vi "PDC_GetStatus.vi"(8 "error in (no error)":errorcluster, 11 "DeviceNo":u32) -> (0 "error out":errorcluster, 2 "Status":u32, 3 "ReturnValue":u32, 4 "ErrorCode":u32)   [LabVIEW 2015]
doc: "This VI retrieves the operating condition of the specified device."
uses:
  PDCLIB.dll
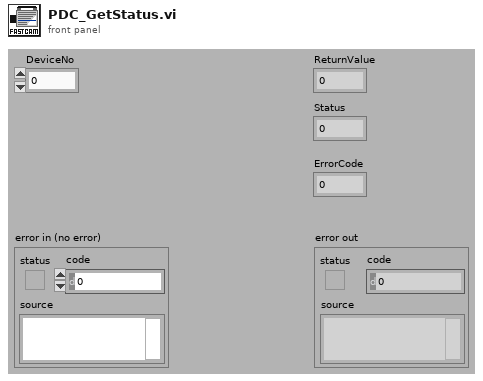
[diagram p1: front panel]
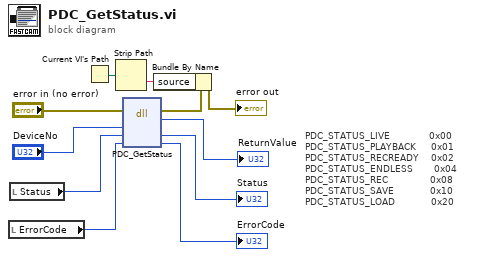
[diagram p0: block diagram]
diagram:
  # "PDC_STATUS_LIVE\t\t\t\t\t\t       0x00\nPDC_STATUS_PLAYBACK\t\t\t\t\t0x01\nPDC_STATUS_RECREADY\t\t\t\t0x02\nPDC_STATUS_ENDLESS\t\t\t\t\t  0x04\nPDC_STATUS_REC\t\t\t\t\t\t        0x08\nPDC_STATUS_SAVE\t\t\t\t\t       0x10\nPDC_STATUS_LOAD\t\t\t\t\t\t      0x20"
  n1 = local read "ErrorCode"() -> (w8:u32)
  n2 = local read "Status"() -> (w6:u32)
  n3 = Current VI's Path() -> (path=w3:path)
  n4 = Strip Path(path=w3) -> (name=w4:string)  [unwired: 1 out]
  n5 = dll-call lib="PDCLIB.dll" fn="PDC_GetStatus"(error in="error in (no error)", "nDeviceNo"="DeviceNo", "pStatus"=w6, "pErrorCode"=w8) -> (error out=w2:errorcluster, "return type"=→"ReturnValue":u32, "pStatus"=→"Status":u32, "pErrorCode"=→"ErrorCode":u32)  [unwired: 3 in, 1 out]
  n6 = Bundle By Name(cluster=w2, "source"=w4) -> (→"error out":errorcluster)
